vi "HarmonicFilterSettings.vi"(0 "Interface in":T2, 5 "HarmonicFilterSettings":cluster{"enable":bool, "coeff":T1}, 9 "timeout (5000 ms)":i32=5000, 11 "error in":errorcluster) -> (4 "Interface out":T2, 15 "error out":errorcluster)   [LabVIEW 2017, in "ThreePhasePLLInterface.lvlib"]
uses:
  ThreePhasePLLInterface.lvlib
  InterfaceRef.ctl
  <instrlib>/_niInstr/Instruction Framework/v1/Host/Instruction Target/niInstr Instruction Target v1 Host.lvclass
  <instrlib>/_niInstr/Instruction Framework/v1/Host/Instruction Framework Context/niInstr Instruction Framework Context v1 Host.lvclass
  FPGA/HarmonicFilter.ctl
  <vilib>/NI/JSON Support for LabVIEW/JSON Data Classes/JSON Object/JSON Object.lvclass
  C:/Program Files (x86)/National Instruments/LabVIEW 2017/vi.lib/NI/JSON Support for LabVIEW/JSON Data Classes/JSON Datatype/JSON Null.lvclass
  <vilib>/NI/JSON Support for LabVIEW/JSON Data Classes/JSON Object/New JSON Object (Empty).vi
  <vilib>/NI/JSON Support for LabVIEW/JSON Data Classes/JSON Object/Insert Key Value Pair (Single).vi
  <vilib>/NI/JSON Support for LabVIEW/JSON Data Classes/JSON Helper/To File (Path).vi
  <vilib>/NI/JSON Support for LabVIEW/JSON Data Classes/JSON Helper/To More Specific Type (Object).vi
  <vilib>/NI/JSON Support for LabVIEW/JSON Data Classes/JSON Helper/JSON Helper.lvclass
  C:/Program Files (x86)/National Instruments/LabVIEW 2017/vi.lib/NI/JSON Support for LabVIEW/JSON Data Classes/JSON Structured Type/JSON Structure.lvclass
  FPGA/ThreePhasePLL.lvlib
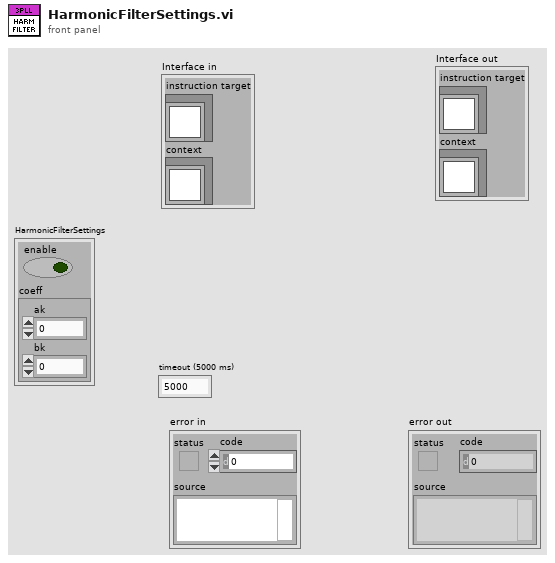
[diagram p1: front panel]
types:
  T1 = typedef "ThreePhasePLL.lvlib/HarmonicFilter.ctl" = cluster{"ak":sgl, "bk":sgl}
  T2 = typedef "ThreePhasePLLInterface.lvlib/InterfaceRef.ctl" = cluster{"instruction target":refnum<class "niInstr Instruction Target v1 Host.lvclass">, "context":refnum<class "niInstr Instruction Framework Context v1 Host.lvclass">}
  T3 = enum16{"open", "replace", "create", "open or create", "replace or create", "replace or create with confirmation"}
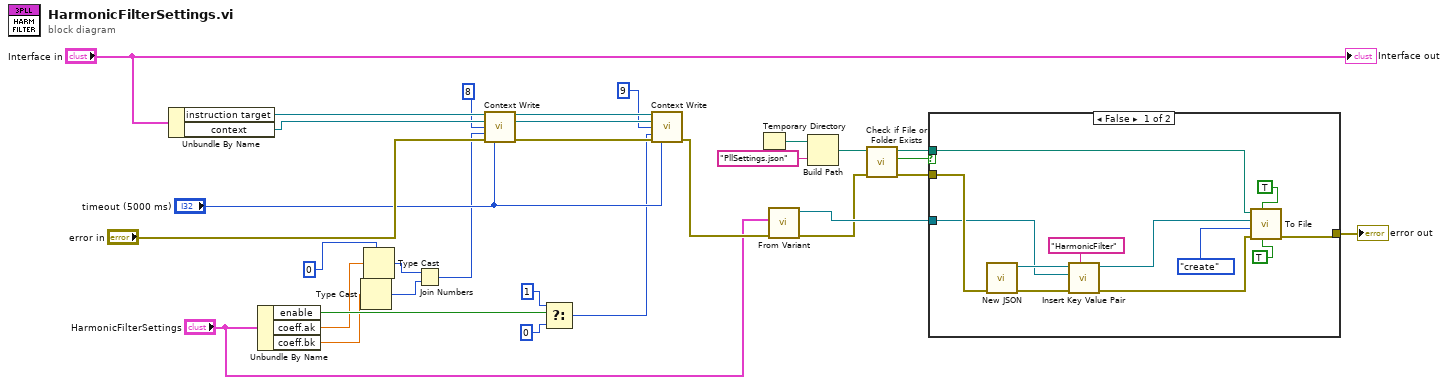
[diagram p0: block diagram]
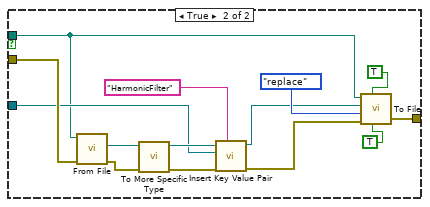
[diagram p2: hidden frame]
diagram:
  w16 = 0
  n1 = Unbundle By Name("Interface in") -> ("instruction target"=w31:refnum<class "niInstr Instruction Target v1 Host.lvclass">, "context"=w30:refnum<class "niInstr Instruction Framework Context v1 Host.lvclass">)
  n2 = Unbundle By Name("HarmonicFilterSettings") -> ("enable"=w25:bool, "coeff.ak"=w18:sgl, "coeff.bk"=w17:sgl)
  n3 = Type Cast(type=w16, x=w17) -> (*(type *) &x=w14:i32)
  n4 = Type Cast(type=w16, x=w18) -> (*(type *) &x=w15:i32)
  n5 = Join Numbers(hi=w15, lo=w14) -> ((hi.lo)=w12:u64)
  n6 = call <instrlib>:"Context Write.vi"("instruction target in"=w31, "context in"=w30, "address"=u64 8, "data"=w12, "error in"="error in", "timeout (5000 ms)"="timeout (5000 ms)") -> ("instruction target out"=w26:refnum<class "niInstr Instruction Target v1 Host.lvclass">, "context out"=w24:refnum<class "niInstr Instruction Framework Context v1 Host.lvclass">, "error out"=w27:errorcluster)  [unwired: 7 in]
  n7 = Select(t=u64 1 ("data"), s=w25, f=u64 0) -> (s? t:f=w19:u64)
  n8 = call <instrlib>:"Context Write.vi"("instruction target in"=w26, "context in"=w24, "address"=u64 9 ("data"), "data"=w19, "error in"=w27, "timeout (5000 ms)"="timeout (5000 ms)") -> ("error out"=w3:errorcluster)  [unwired: 7 in, 2 out]
  n9 = Temporary Directory() -> (w10:path)
  n10 = call <vilib>:"From Variant.vi"("error in (no error)"=w3, "Variant"="HarmonicFilterSettings") -> ("error out"=w7:errorcluster, "JSON out"=w11:refnum<class "JSON Null.lvclass">)  [unwired: 8 in]
  n11 = Build Path(base path=w10, name or relative path="PllSettings.json") -> (appended path=w8:path)
  n12 = call <vilib>:"Check if File or Folder Exists.vi"("error in (no error)"=w7, "path"=w8) -> ("error out"=w6:errorcluster, "file or folder exists?"=w1:bool, "dup path"=w5:path)  [unwired: 7 in]
  n13 = case shown="False" w1 {
    tunnel: w11 -> [w35 w49]
    tunnel: w6 -> [w38 w53]
    tunnel: w5 -> [w41 w45]
    tunnel: [w39 w54] -> w4
    frame False {
      n14 = call-poly <vilib>:"New JSON.vi"("error in (no error)"=w38) -> ("error out"=w37:errorcluster, "JSON Object out"=w36:refnum<class "JSON Object.lvclass">)  [unwired: 9 in]
      n15 = call-poly <vilib>:"Insert Key Value Pair.vi"("key"="HarmonicFilter", "error in (no error)"=w37, "value"=w35, "JSON Object in"=w36) -> ("error out"=w33:errorcluster, "JSON Object out"=w32:refnum<class "JSON Object.lvclass">)  [unwired: 5 in, 1 out]
      n16 = call-poly <vilib>:"To File.vi"("Pretty Print?"=TRUE, "enable LabVIEW extensions? (T)"=TRUE, "error in (no error)"=w33, "operation (0:open)"=T3."create", "JSON Datatype in"=w32, "file path"=w41) -> ("error out"=w39:errorcluster)  [unwired: 5 in]
    }
    frame True {
      n17 = call <vilib>:"From File.vi"("error in"=w53, "file path"=w45) -> ("error out"=w51:errorcluster, "JSON out"=w52:refnum<class "JSON Null.lvclass">)  [unwired: 8 in]
      n18 = call-poly <vilib>:"To More Specific Type.vi"("error in (no error)"=w51, "JSON Datatype in"=w52) -> ("error out"=w47:errorcluster, "JSON Datatype out"=w50:refnum<class "JSON Object.lvclass">)  [unwired: 8 in]
      n19 = call-poly <vilib>:"Insert Key Value Pair.vi"("key"="HarmonicFilter", "error in (no error)"=w47, "value"=w49, "JSON Object in"=w50) -> ("error out"=w44:errorcluster, "JSON Object out"=w46:refnum<class "JSON Object.lvclass">)  [unwired: 5 in, 1 out]
      n20 = call-poly <vilib>:"To File.vi"("Pretty Print?"=TRUE, "enable LabVIEW extensions? (T)"=TRUE, "error in (no error)"=w44, "operation (0:open)"=T3."replace", "JSON Datatype in"=w46, "file path"=w45) -> ("error out"=w54:errorcluster)  [unwired: 5 in]
    }
  }
  "error out" <- w4
  "Interface out" <- "Interface in"
